vi "Set Speed.vi"(8 "error in (no error)":errorcluster, 10 "Pump %":sgl, 11 "ASIA Pump C Settings in":T1) -> (0 "error out":errorcluster, 1 "Connection Error":bool, 3 "ASIA Pump C Settings out":T1)   [LabVIEW 2018, in "ASIA Pump.lvlib"]
uses:
  ASIA Pump.lvlib
  Pump Settings.ctl
  Program Files (x86)/Pfizer/FAST/data/AsiaPumpInterface.dll
panel:
  out "Status Connection Error":bool
  out "Task Completed":bool
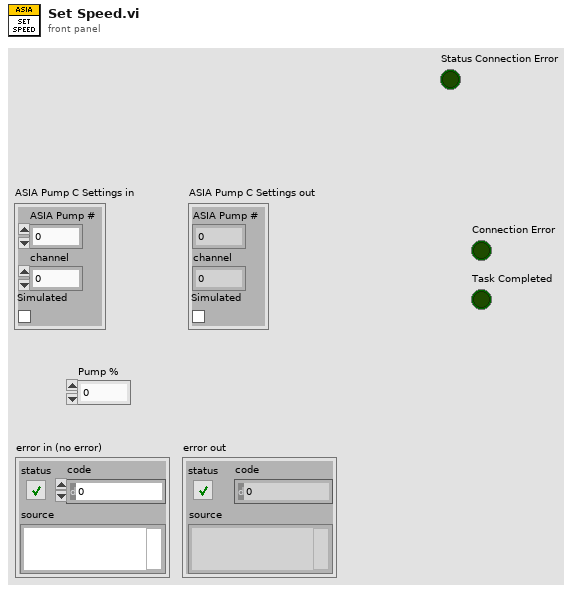
[diagram p1: front panel]
types:
  T1 = typedef "ASIA Pump.lvlib/Pump Settings.ctl" = cluster{"ASIA Pump #":i32, "channel":i32, "Simulated":bool}
  T2 = enum16{"Error", "Uninitialised", "Initialising", "Idle", "Filling", "Full", "Emptying", "Empty", "Pumping", "Default"}
  T3 = cluster{"Busy":bool, "PumpCnt":dbl, "RemoteEntered":bool, "OverpressureSet":bool}[]
  T4 = cluster{"Busy":bool, "PumpCnt":dbl, "RemoteEntered":bool, "OverpressureSet":bool}
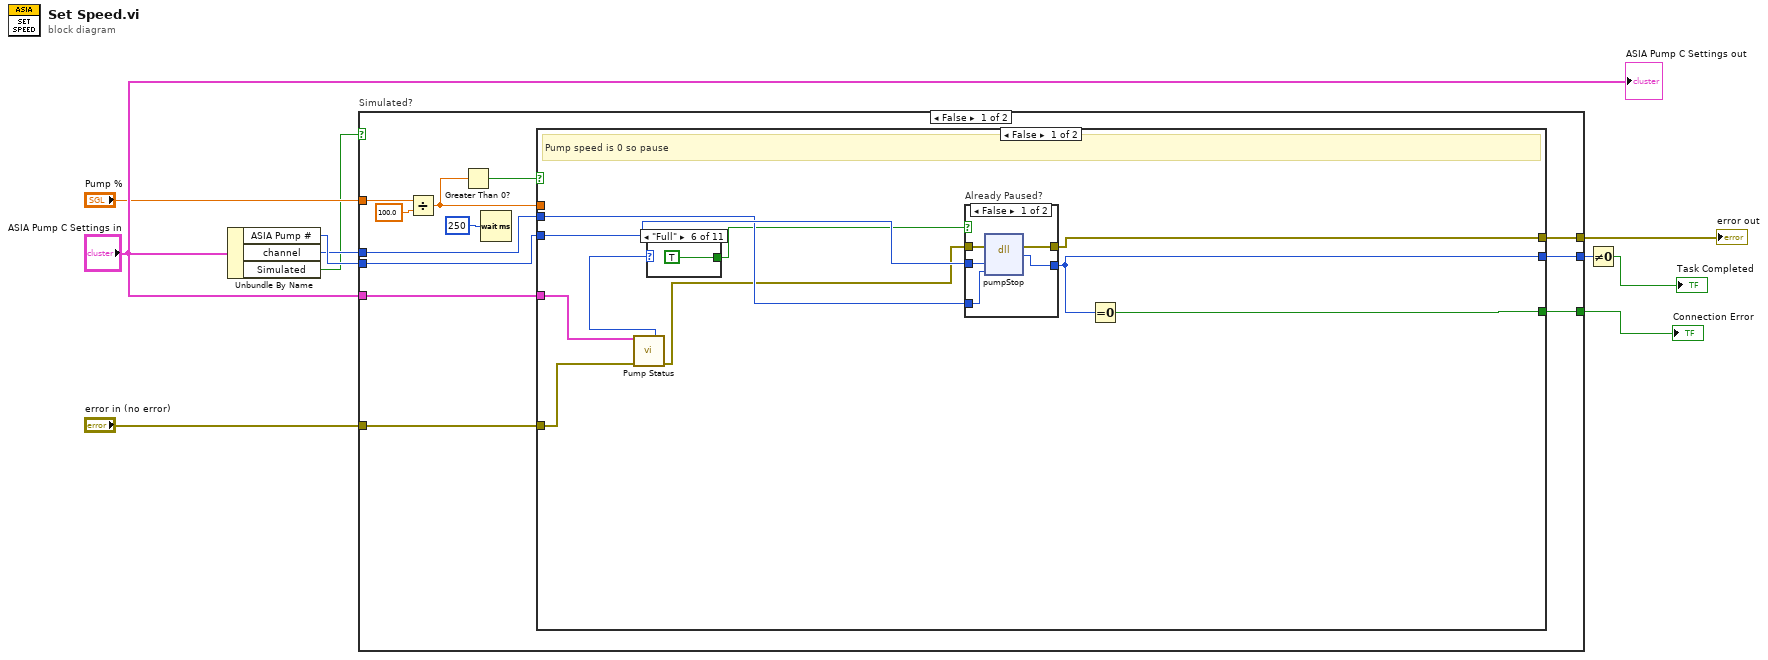
[diagram p0: block diagram]
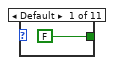
[diagram p2: hidden frame]
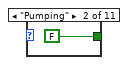
[diagram p3: hidden frame]
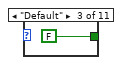
[diagram p4: hidden frame]
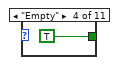
[diagram p5: hidden frame]
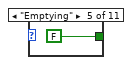
[diagram p6: hidden frame]
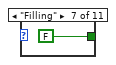
[diagram p7: hidden frame]
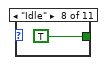
[diagram p8: hidden frame]
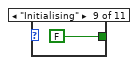
[diagram p9: hidden frame]
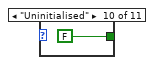
[diagram p10: hidden frame]
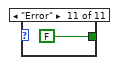
[diagram p11: hidden frame]
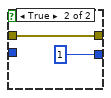
[diagram p12: hidden frame]
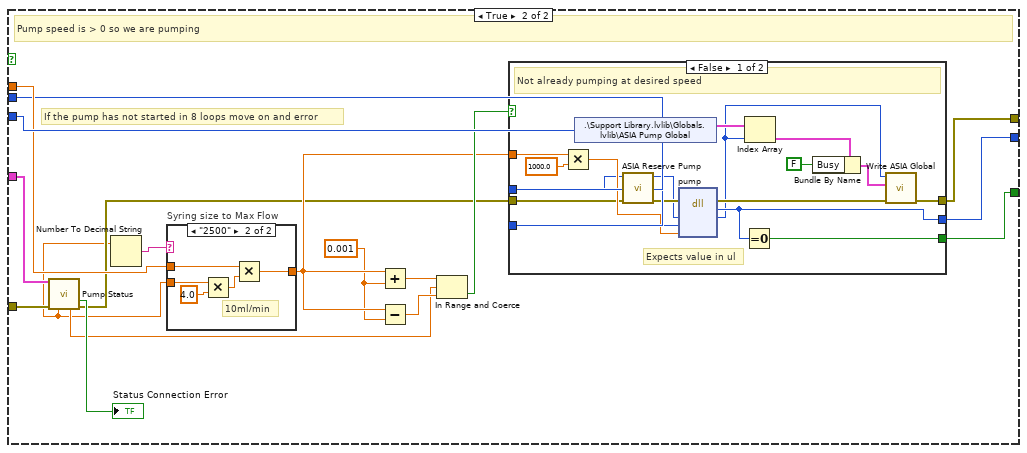
[diagram p13: hidden frame]
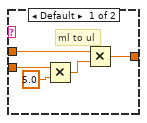
[diagram p14: hidden frame]
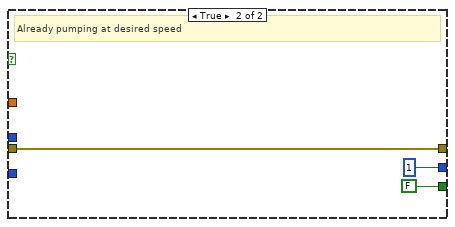
[diagram p15: hidden frame]
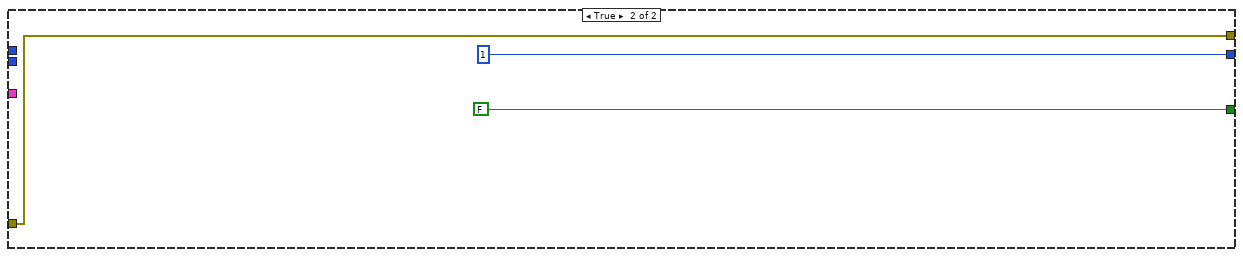
[diagram p16: hidden frame]
diagram:
  n1 = Unbundle By Name("ASIA Pump C Settings in") -> ("ASIA Pump #"=w4:i32, "channel"=w3:i32, "Simulated"=w1:bool)
  n2 = case "Simulated?" shown="False" w1 {
    tunnel: [w22 w101] -> w9
    tunnel: "ASIA Pump C Settings in" -> [w21 _]
    tunnel: "error in (no error)" -> [w20 w101]
    tunnel: w4 -> [w19 _]
    tunnel: w3 -> [w18 _]
    tunnel: [w17 FALSE ("Connection Error")] -> w6
    tunnel: [w16 1 ("Bool")] -> w2
    tunnel: "Pump %" -> [w14 _]
    frame False {
      n3 = Divide(x=w14, y=sgl 100.0) -> (x/y=w13:sgl)
      n4 = Greater Than 0?(x=w13) -> (x > 0?=w12:bool)
      n5 = Wait (ms)(milliseconds to wait=u32 250) -> ()  [unwired: 1 out]
      n6 = case shown="False" w12 {
        tunnel: [w30 w58] -> w22
        tunnel: w19 -> [w32 w68]
        tunnel: w18 -> [w31 w57]
        tunnel: w13 -> [_ w65]
        tunnel: [w28 w67] -> w17
        tunnel: [w27 w66] -> w16
        tunnel: w20 -> [w24 w56]
        tunnel: w21 -> [w26 w55]
        frame False {
          # "Pump speed is 0 so pause"
          n7 = call "Pump Status.vi"("ASIA Pump C Settings in"=w26, "error in (no error)"=w24) -> ("PumpStatusCode"=w25:T2, "error out"=w23:errorcluster)  [unwired: 5 in, 7 out]
          n8 = case shown="\"Full\"" w25 {
            tunnel: [FALSE FALSE FALSE TRUE FALSE TRUE FALSE TRUE FALSE FALSE FALSE] -> w29
            frame Default {
            }
            frame "Pumping" {
            }
            frame "Default" {
            }
            frame "Empty" {
            }
            frame "Emptying" {
            }
            frame "Full" {
            }
            frame "Filling" {
            }
            frame "Idle" {
            }
            frame "Initialising" {
            }
            frame "Uninitialised" {
            }
            frame "Error" {
            }
          }
          n9 = case "Already Paused?" shown="False" w29 {
            tunnel: w32 -> [w48 _]
            tunnel: w31 -> [w47 _]
            tunnel: [w46 1 ("Bool")] -> w27
            tunnel: [w45 w50] -> w30
            tunnel: w23 -> [w44 w50]
            frame False {
              n10 = dll-call lib="C:/Program Files (x86)/Pfizer/FAST/data/AsiaPumpInterface.dll" fn="pumpStop"(error in=w44, "pumpNum"=w48, "channel"=w47) -> (error out=w45:errorcluster, "Bool"=w46:u8)  [unwired: 4 in, 1 out]
            }
            frame True {
            }
          }
          n11 = Equal To 0?(x=w27) -> (x = 0?=w28:bool)
        }
        frame True {
          w61 = 0.001 ("y")
          # "If the pump has not started in 8 loops move on and error"
          # "Pump speed is > 0 so we are pumping"
          n12 = call "Pump Status.vi"("ASIA Pump C Settings in"=w55, "error in (no error)"=w56) -> ("Connection Error"=→"Status Connection Error":bool, "syringeSize (ml)"=w51:sgl, "pumpRate"=w52:dbl, "error out"=w53:errorcluster)  [unwired: 5 in, 5 out]
          n13 = Number To Decimal String(number=w51) -> (decimal integer string=w64:string)  [unwired: 1 in]
          n14 = case "Syring size to Max Flow" shown="\"2500\"" w64 {
            tunnel: w65 -> [w71 w75]
            tunnel: [w69 w74] -> w62
            tunnel: w51 -> [w70 w78]
            frame Default {
              # "ml to ul"
              n15 = Multiply(x=w70, y=5.0) -> (x*y=w73:dbl)
              n16 = Multiply(x=w71, y=w73) -> (x*y=w69:dbl)
            }
            frame "2500" {
              # "10ml/min"
              n17 = Multiply(x=w78, y=sgl 4.0) -> (x*y=w76:sgl)
              n18 = Multiply(x=w75, y=w76) -> (x*y=w74:sgl)
            }
          }
          n19 = Add(x=w62, y=w61) -> (x+y=w60:dbl)
          n20 = Subtract(x=w62, y=w61) -> (x-y=w59:dbl)
          n21 = In Range and Coerce(upper limit=w60, x=w52, lower limit=w59) -> (In Range?=w63:bool)  [unwired: 1 out]
          n22 = case shown="False" w63 {
            tunnel: w68 -> [w87 _]
            tunnel: w57 -> [w95 _]
            tunnel: w62 -> [w91 _]
            tunnel: [w94 FALSE] -> w67
            tunnel: w53 -> [w89 w96]
            tunnel: [w93 u8 1 ("Bool")] -> w66
            tunnel: [w84 w96] -> w58
            frame False {
              # "Expects value in ul"
              # "Not already pumping at desired speed"
              n23 = Multiply(x=w91, y=1000.0) -> (x*y=w90:dbl)
              n24 = shared-variable ".\\Support Library.lvlib\\Globals.lvlib\\ASIA Pump Global"() -> (w81:T3)  [unwired: 1 in, 1 out]
              n25 = call "ASIA Reserve Pump.vi"("error in (no error)"=w89, "ASIA Pump #"=w87) -> ("error out"=w88:errorcluster, "ASIA Pump #"=w86:i32)  [unwired: 8 in]
              n26 = dll-call lib="C:/Program Files (x86)/Pfizer/FAST/data/AsiaPumpInterface.dll" fn="pump"(error in=w88, "pumpNum"=w86, "channel"=w95, "rate"=w90) -> (error out=w85:errorcluster, "Bool"=w93:u8, "pumpNum"=w79:u32)  [unwired: 4 in, 1 out]
              n27 = Equal To 0?(x=w93) -> (x = 0?=w94:bool)
              n28 = Index Array(array=w81, index=w79) -> (element=w80:T4)
              n29 = Bundle By Name(cluster=w80, "Busy"=FALSE) -> (w82:T4)
              n30 = call "Write ASIA Global.vi"("error in (no error)"=w85, "ASIA Global"=w82, "Pump Number"=w79) -> ("error out"=w84:errorcluster)  [unwired: 7 in, 1 out]
            }
            frame True {
              # "Already pumping at desired speed"
            }
          }
        }
      }
    }
    frame True {
    }
  }
  "Connection Error" <- w6
  "error out" <- w9
  n31 = Not Equal To 0?(x=w2) -> (x != 0?=→"Task Completed":bool)
  "ASIA Pump C Settings out" <- "ASIA Pump C Settings in"
